vi "Read Setting.vi"(8 "error in (no error)":errorcluster, 11 "Update SGL Array in":refnum<class "Update SGL Array.lvclass">) -> (0 "error out":errorcluster, 2 "Setting":sgl[](array[numeric]), 3 "Update SGL Array out":refnum<class "Update SGL Array.lvclass">)   [LabVIEW 2014, in "Update SGL Array.lvclass"]
uses:
  Update SGL Array.lvclass
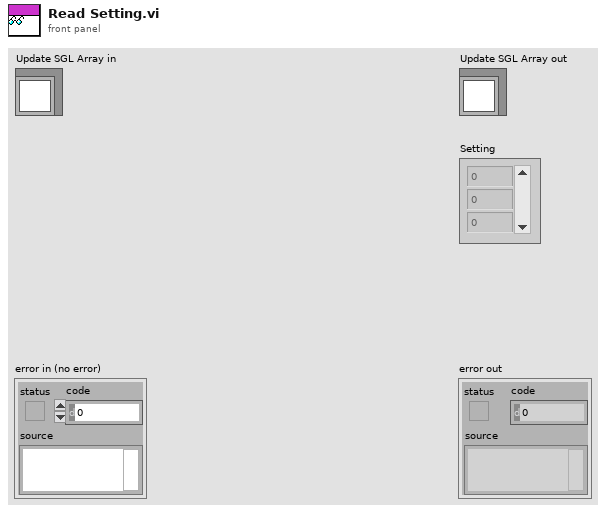
[diagram p1: front panel]
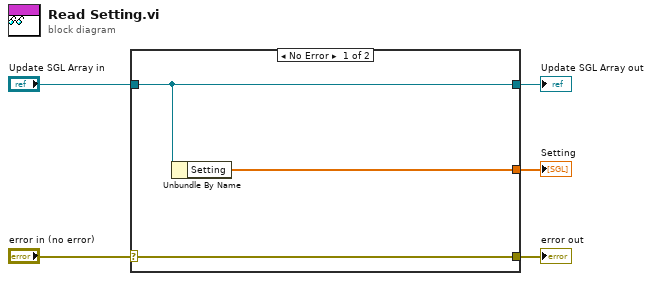
[diagram p0: block diagram]
diagram:
  n1 = case shown="No Error" "error in (no error)" {
    selector: "error in (no error)" -> [w8 w9]
    tunnel: [w8 w9] -> w4
    tunnel: [w7 w10] -> w2
    tunnel: "Update SGL Array in" -> [w7 w10]
    tunnel: [w6 _] -> w1
    frame No Error {
      n2 = Unbundle By Name(w7) -> ("Setting"=w6:sgl[])
    }
    frame Error {
    }
  }
  "error out" <- w4
  "Update SGL Array out" <- w2
  "Setting" <- w1
